vi "SRV_Append Filename Extension if Necessary.vi"(5 "Filename":string, 9 "Extension":string) -> (8 "Filename with Extension":string)   [LabVIEW 2014]
doc: "Appends Extension to Filename if the specified extension is not already the end of Filename.\n\n\nAuthor: Mike Schultz"
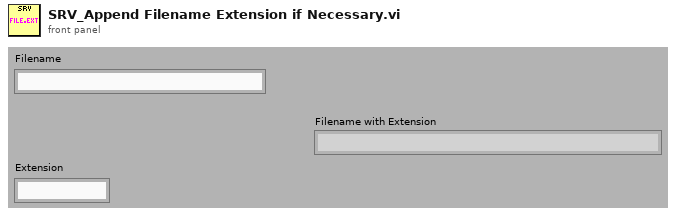
[diagram p1: front panel]
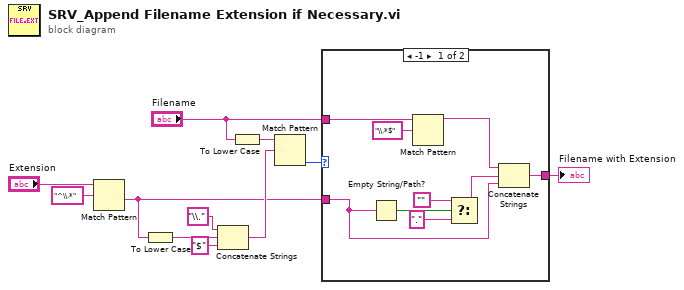
[diagram p0: block diagram]
diagram:
  n1 = Match Pattern(string="Extension", regular expression="^\\.*") -> (after substring=w1:string)  [unwired: 4 out]
  n2 = To Lower Case(string=w1) -> (all lower case string=w11:string)
  n3 = Concatenate Strings("\\." ("string"), w11, "$" ("string")) -> (w8:string)
  n4 = To Lower Case(string="Filename") -> (all lower case string=w4:string)
  n5 = Match Pattern(string=w4, regular expression=w8) -> (offset past match=w7:i32)  [unwired: 4 out]
  n6 = case shown="-1" w7 {
    tunnel: "Filename" -> [w14 w21]
    tunnel: w1 -> [w16 _]
    tunnel: [w20 w21] -> w5
    frame -1 {
      n7 = Empty String/Path?(string/path=w16) -> (empty?=w19:bool)
      n8 = Match Pattern(string=w14, regular expression="\\.*$") -> (before substring=w13:string)  [unwired: 4 out]
      n9 = Select(t="", s=w19, f="." ("y")) -> (s? t:f=w17:string)
      n10 = Concatenate Strings(w13, w17, w16) -> (w20:string)
    }
    frame Default {
    }
  }
  "Filename with Extension" <- w5
